vi "GLVT-Stepper-HWInteract.vi"(7 "GLVT-Enable State":T1, 8 "error in":errorcluster, 9 "Direction (T=CW)":bool, 10 "Pulse":bool) -> (0 "error out":errorcluster)   [LabVIEW 2020]
uses:
  Controls/GLVT-Stepper-EnableState.ctl
  <vilib>/DAQmx/write.llb/DAQmx Write (Digital 1D Bool NChan 1Samp 1Line).vi
  <vilib>/DAQmx/miscellaneous.llb/DAQmx Fill In Error Info.vi
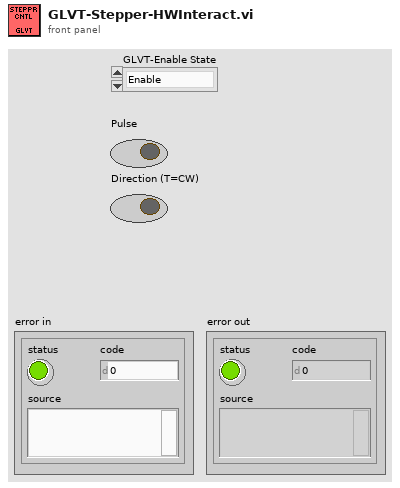
[diagram p1: front panel]
types:
  T1 = typedef "GLVT-Stepper-EnableState.ctl" = enum16{"Enable", "Disable"}
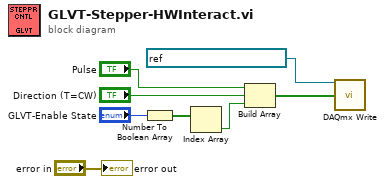
[diagram p0: block diagram]
diagram:
  n1 = Number To Boolean Array(number="GLVT-Enable State") -> (Boolean array=w5:bool[])
  n2 = Index Array(array=w5) -> (element=w2:bool)  [unwired: 1 in]
  n3 = Build Array("Pulse", "Direction (T=CW)", w2) -> (w3:bool[])
  n4 = call-poly <vilib>:"DAQmx Write.vi"("task/channels in"=refnum<k21> "GLVT-StepperControl", "data"=w3) -> ()  [unwired: 11 in, 3 out]
  "error out" <- "error in"
